vi "Load settings from backup.vi"(6 "Enable":bool, 8 "error in (no error)":errorcluster, 9 "file path (dialog if empty)":path, 10 "Cluster in":T1, 11 "VISA Refnum in":refnum<visa-resource-name>) -> (0 "error out":errorcluster, 2 "Cluster out":T1, 3 "VISA Refnum out":refnum<visa-resource-name>)   [LabVIEW 2020]
uses:
  82bf5f74-efaa-45ba-9adc-4a4c24cd7e01.vi
  ae98ab40-b3fa-4478-8993-6b4b5b607684.vi
  47921e7e-a47f-465c-9279-a097ef6c73d7.vi
  <vilib>/Utility/file.llb/Read Delimited Spreadsheet (string).vi
  WriteSingleCoil.vi
  <vilib>/NI Modbus.llb/MB Serial Master Query (poly).vi
  <vilib>/NI Modbus.llb/MB Serial Master Query Write Single Register (poly).vi
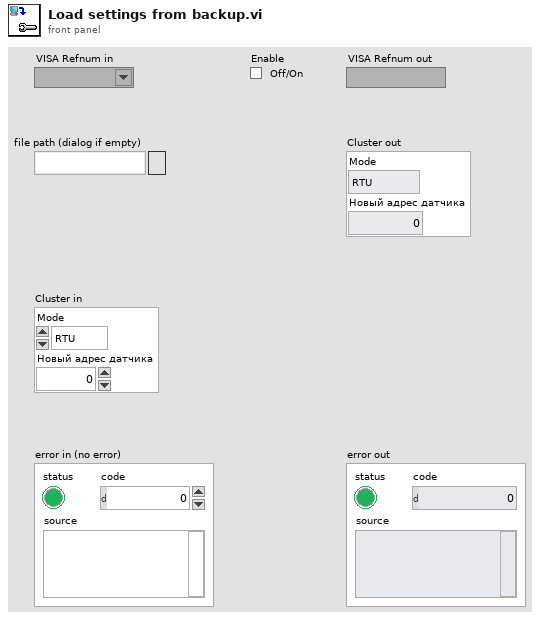
[diagram p1: front panel]
types:
  T1 = cluster{"Mode":enum16{"RTU", "ASCII"}, "Новый адрес датчика":u16}
  T2 = cluster{"Name":string, "Address":u16, "Type":u16, "Value":sgl}
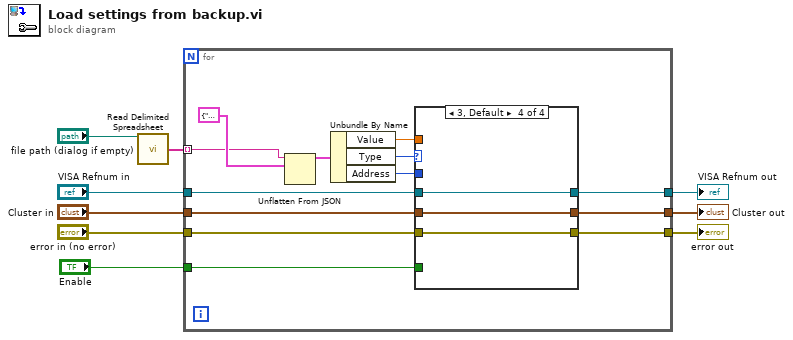
[diagram p0: block diagram]
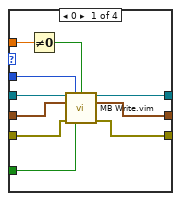
[diagram p2: hidden frame]
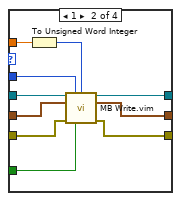
[diagram p3: hidden frame]
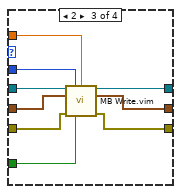
[diagram p4: hidden frame]
diagram:
  n1 = call-poly <vilib>:"Read Delimited Spreadsheet.vi"("file path (dialog if empty)"="file path (dialog if empty)") -> ("first row"=w1:string[])  [unwired: 9 in, 5 out]
  n2 = for {
    tunnel: w1 -> [w21] mode=indexing
    tunnel: "VISA Refnum in" -> [w16]
    tunnel: "Cluster in" -> [w15]
    tunnel: "error in (no error)" -> [w14]
    tunnel: [w13] -> w5
    tunnel: [w12] -> w6
    tunnel: [w11] -> w7
    tunnel: "Enable" -> [w10]
    n3 = Unflatten From JSON(JSON string=w21, type and defaults=T2 {"Name"="", "Address"=0, "Type"=0, "Value"=0.0}) -> (value=w20:T2)  [unwired: 5 in, 1 out]
    n4 = Unbundle By Name(w20) -> ("Value"=w17:sgl, "Type"=w19:u16, "Address"=w18:u16)
    n5 = case shown="3, Default" w19 {
      tunnel: w18 -> [w32 w42 w51 _]
      tunnel: w17 -> [w31 w41 w50 _]
      tunnel: w16 -> [w29 w39 w49 w54]
      tunnel: w15 -> [w28 w38 w47 w53]
      tunnel: w14 -> [w27 w37 w45 w52]
      tunnel: [w26 w36 w48 w54] -> w13
      tunnel: [w25 w35 w46 w53] -> w12
      tunnel: [w24 w34 w44 w52] -> w11
      tunnel: w10 -> [w23 w33 w43 _]
      frame 0 {
        n6 = Not Equal To 0?(x=w31) -> (x != 0?=w30:bool)
        n7 = call "MB Write.vim"("VISA Refnum in"=w29, "Command"=w32, "Data"=w30, "Cluster"=w28, "error in"=w27, "Enable"=w23) -> ("VISA out"=w26:refnum<visa-resource-name>, "Cluster Out"=w25:T1, "error out"=w24:errorcluster)  [unwired: 7 in]
      }
      frame 1 {
        n8 = To Unsigned Word Integer(number=w41) -> (unsigned 16bit integer=w40:u16)
        n9 = call "MB Write.vim"("VISA Refnum in"=w39, "Command"=w42, "Data"=w40, "Cluster"=w38, "error in"=w37, "Enable"=w33) -> ("VISA out"=w36:refnum<visa-resource-name>, "Cluster Out"=w35:T1, "error out"=w34:errorcluster)  [unwired: 7 in]
      }
      frame 2 {
        n10 = call "MB Write.vim"("VISA Refnum in"=w49, "Command"=w51, "Data"=w50, "Cluster"=w47, "error in"=w45, "Enable"=w43) -> ("VISA out"=w48:refnum<visa-resource-name>, "Cluster Out"=w46:T1, "error out"=w44:errorcluster)  [unwired: 7 in]
      }
      frame 3, Default {
      }
    }
  }
  "error out" <- w7
  "Cluster out" <- w6
  "VISA Refnum out" <- w5
